vi "configure.vi"(8 "error in (no error)":errorcluster, 9 "Value":i32, 10 "ILC":refnum<class "ILC.lvclass">, 11 "IConfigureILCStrategy in":refnum<class "ConfigureILCDAC4Strategy.lvclass">) -> (0 "error out":errorcluster, 3 "IConfigureILCStrategy out":refnum<class "ConfigureILCDAC4Strategy.lvclass">)   [LabVIEW 2015, in "ConfigureILCDAC4Strategy.lvclass"]
uses:
  ConfigureILCDAC4Strategy.lvclass
  <userlib>/Common/ILC/ILC/ILC.lvclass
  <userlib>/Common/ILC/ILC/ILC.lvclass/ILC.ctl
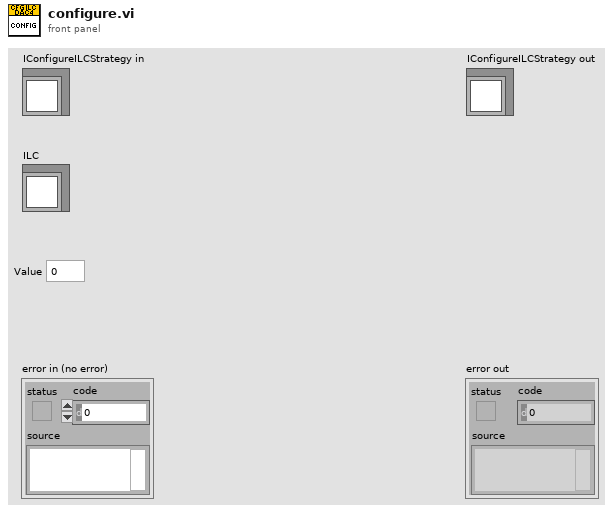
[diagram p1: front panel]
types:
  T1 = typedef "ILCCommon.lvlib/ILCTypedefs.lvlib/OutputData.ctl" = cluster{"Step & Direction":i16, "Blower RPM":u8, "PWM (SSR)":u8, "Ch1":u16, "Ch2":u16, "Ch3":u16, "Ch4":u16}
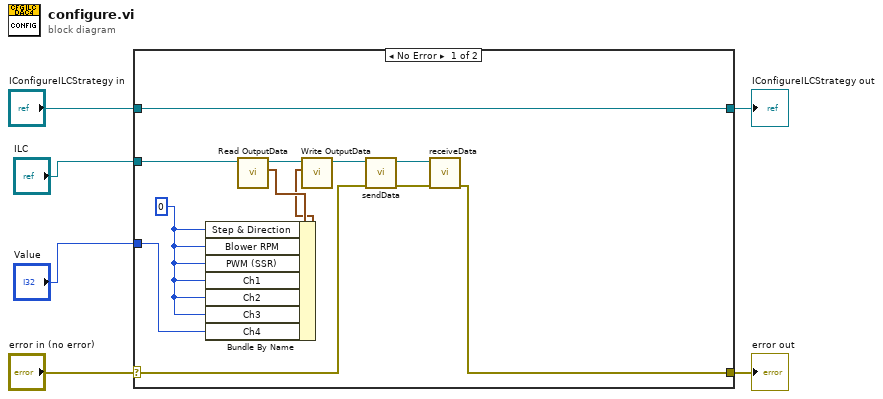
[diagram p0: block diagram]
diagram:
  n1 = case shown="No Error" "error in (no error)" {
    selector: "error in (no error)" -> [w13 w20]
    tunnel: [w11 w20] -> w5
    tunnel: [w18 w19] -> w3
    tunnel: "IConfigureILCStrategy in" -> [w18 w19]
    tunnel: "ILC" -> [w17 _]
    tunnel: "Value" -> [w7 _]
    frame No Error {
      w10 = i16 0 ("Step & Direction")
      n2 = call <userlib>:"Read OutputData.vi"("ILC in"=w17) -> ("OutputData"=w9:T1, "ILC out"=w16:refnum<class "ILC.lvclass">)  [unwired: 9 in]
      n3 = Bundle By Name(cluster=w9, "Step & Direction"=w10, "Blower RPM"=w10, "PWM (SSR)"=w10, "Ch1"=w10, "Ch2"=w10, "Ch3"=w10, "Ch4"=w7) -> (w8:T1)
      n4 = call <userlib>:"Write OutputData.vi"("OutputData"=w8, "ILC in"=w16) -> ("ILC out"=w15:refnum<class "ILC.lvclass">)  [unwired: 9 in]
      n5 = call <userlib>:"sendData.vi"("error in (no error)"=w13, "ILC in"=w15) -> ("error out"=w12:errorcluster, "ILC out"=w14:refnum<class "ILC.lvclass">)  [unwired: 8 in]
      n6 = call <userlib>:"receiveData.vi"("error in (no error)"=w12, "ILC in"=w14) -> ("error out"=w11:errorcluster)  [unwired: 8 in, 1 out]
    }
    frame Error {
    }
  }
  "error out" <- w5
  "IConfigureILCStrategy out" <- w3
